vi "GetAsyncDVR.vi"(8 "error in (no error)":errorcluster, 11 "MicronGRPCClient in":refnum<class "MicronGRPCClient.lvclass">) -> (0 "error out":errorcluster, 2 "AsyncDVR":refnum<data-value>, 3 "MicronGRPCClient out":refnum<class "MicronGRPCClient.lvclass">)   [LabVIEW 2019, in "MicronGRPCClient.lvclass"]
uses:
  MicronGRPCClient.lvclass
  Typedefs/AsyncCluster.ctl
  <vilib>/SLL Toolkit/SLL Queued State Machine/Queue Driver/Typedefs/Queue Type.ctl
  <vilib>/gRPC/LabVIEW gRPC Library/Shared/grpcId.ctl
  MicronGRPCClient.lvclass/MicronGRPCClient.ctl
  <vilib>/SLL Toolkit/SLL Queued State Machine/Queue Driver/Create Queue.vi
  <vilib>/SLL Toolkit/SLL Queued State Machine/SLL QSM.lvlib
  <vilib>/gRPC/LabVIEW gRPC Library/grpc-lvsupport-release.lvlib
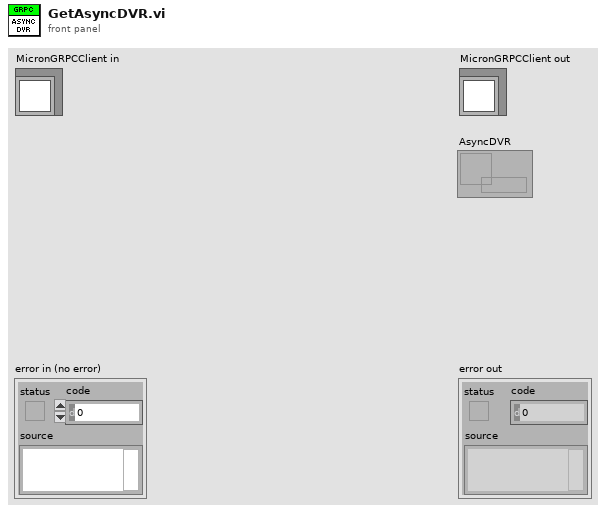
[diagram p1: front panel]
types:
  T1 = typedef "MicronGRPCClient.lvclass/AsyncCluster.ctl" = cluster{"QueueRef":refnum<queue>, "PackageName":string, "ServiceName":string, "gRPC ID":T2, "Simulate?":bool}
  T2 = typedef "grpc-lvsupport-release.lvlib/grpcId.ctl" = u64
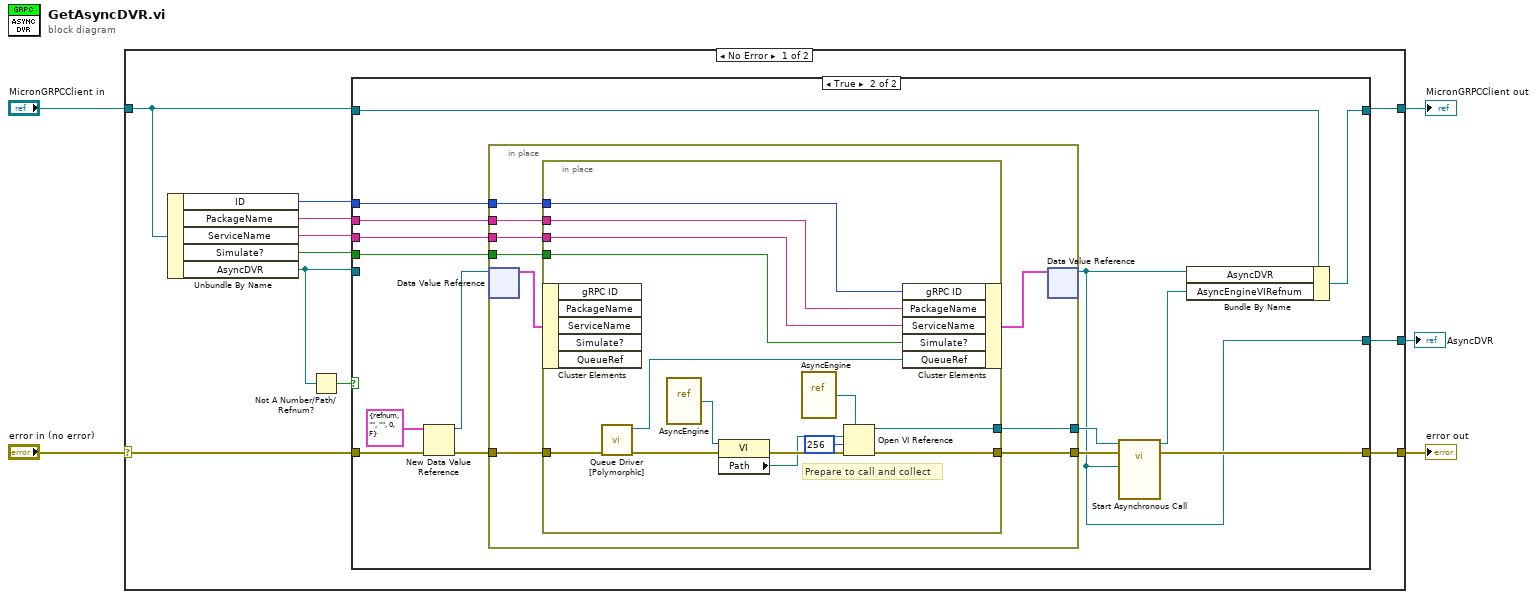
[diagram p0: block diagram]
diagram:
  n1 = case shown="No Error" "error in (no error)" {
    selector: "error in (no error)" -> [w15 w58]
    tunnel: [w16 w58] -> w4
    tunnel: [w7 w57] -> w2
    tunnel: "MicronGRPCClient in" -> [w8 w57]
    tunnel: [w6 _] -> w1
    frame No Error {
      n2 = Unbundle By Name(w8) -> ("ID"=w10:T2, "PackageName"=w11:string, "ServiceName"=w12:string, "Simulate?"=w9:bool, "AsyncDVR"=w13:refnum<data-value>)
      n3 = Not A Number/Path/Refnum?(number/path/refnum=w13) -> (NaN/Path/Refnum?=w14:bool)
      n4 = case shown="True" w14 {
        tunnel: [w18 w23] -> w16
        tunnel: w15 -> [w18 w32]
        tunnel: w13 -> [_ _]
        tunnel: w12 -> [_ w31]
        tunnel: w11 -> [_ w30]
        tunnel: w10 -> [_ w29]
        tunnel: w9 -> [_ w28]
        tunnel: w8 -> [w17 w21]
        tunnel: [w17 w20] -> w7
        tunnel: [_ w19] -> w6
        frame False {
        }
        frame True {
          n5 = New Data Value Reference(data value=T1 {"QueueRef"=refnum, "PackageName"="", "ServiceName"="", "gRPC ID"=0, "Simulate?"=FALSE} ("Async"), error in=w32) -> (data value reference=w26:refnum<data-value>, error out=w33:errorcluster)
          n6 = in-place {
            in-place-border: [w42] -> w24
            in-place-border: w33 -> [w41]
            in-place-border: w31 -> [w38]
            in-place-border: w30 -> [w37]
            in-place-border: w29 -> [w36]
            in-place-border: w28 -> [w35]
            in-place-border: [w34] -> w25
            n7 = in-place-dvr #1(w26) -> (w40:T1)  [unwired: 1 out]
            n8 = in-place {
              in-place-border: [w43] -> w42
              in-place-border: w41 -> [w55]
              in-place-border: w38 -> [w50]
              in-place-border: w37 -> [w49]
              in-place-border: w36 -> [w48]
              in-place-border: w35 -> [w47]
              in-place-border: [w44] -> w34
              # "Prepare to call and collect"
              n9 = in-place-cluster #2(w40) -> ()  [unwired: 5 out]
              n10 = call-poly <vilib>:"Queue Driver [Polymorphic].vi"("Error In"=w55) -> ("Error Out"=w56:errorcluster, "Queue Ref"=w52:refnum<queue>)  [unwired: 9 in]
              n11 = vi-ref "AsyncEngine.vi"() -> (w51:refnum<vi>)
              n12 = property class="VI"(reference=w51, error in=w56) -> (error out=w54:errorcluster, "Path"=w53:path)  [unwired: 1 out]
              n13 = vi-ref "AsyncEngine.vi"() -> (w45:refnum<vi>)
              n14 = Open VI Reference(type specifier VI Refnum (for type only)=w45, vi path=w53, options=256, error in (no error)=w54) -> (vi reference=w44:refnum<vi>, error out=w43:errorcluster)  [unwired: 2 in]
              n15 = in-place-cluster #2("gRPC ID"=w48, "PackageName"=w49, "ServiceName"=w50, "Simulate?"=w47, "QueueRef"=w52) -> (w39:T1)
            }
            n16 = in-place-dvr #1(w39) -> (w19:refnum<data-value>)  [unwired: 1 out]
          }
          n17 = call-by-ref "Start Asynchronous Call"(reference=w25, error in=w24, "AsyncDVR"=w19) -> (reference out=w22:refnum<vi>, error out=w23:errorcluster)  [unwired: 10 in, 1 out]
          n18 = Bundle By Name(cluster=w21, "AsyncDVR"=w19, "AsyncEngineVIRefnum"=w22) -> (w20:refnum<class "MicronGRPCClient.lvclass">)
        }
      }
    }
    frame Error {
    }
  }
  "error out" <- w4
  "MicronGRPCClient out" <- w2
  "AsyncDVR" <- w1
